vi "IE_Open Help Link.vi"(8 "error in (no error)":errorcluster, 11 "Help.URL":string) -> (0 "error out":errorcluster)   [LabVIEW 2021]
uses:
  <vilib>/Platform/browser.llb/Open URL in Default Browser (string).vi
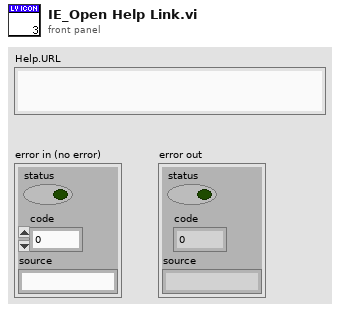
[diagram p1: front panel]
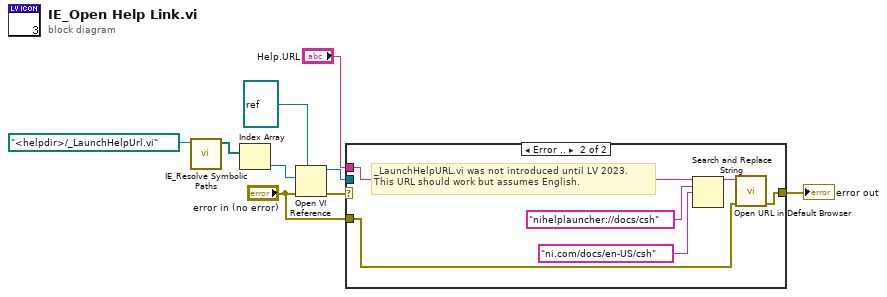
[diagram p0: block diagram]
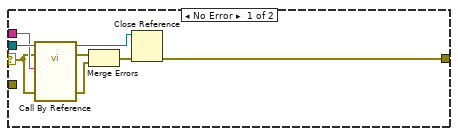
[diagram p2: hidden frame]
diagram:
  n1 = call "IE_Resolve Symbolic Paths.vi"("symbolic path"=path "<helpdir>/_LaunchHelpUrl.vi") -> ("resolved paths"=w8:path[])  [unwired: 10 in]
  n2 = Index Array(array=w8) -> (element=w7:path)  [unwired: 1 in]
  n3 = Open VI Reference(type specifier VI Refnum (for type only)=refnum<vi> refnum, vi path=w7, error in (no error)="error in (no error)") -> (vi reference=w6:refnum<vi>, error out=w3:errorcluster)  [unwired: 3 in]
  n4 = case shown="Error .." w3 {
    selector: w3 -> [w15 _]
    tunnel: w6 -> [w17 _]
    tunnel: "Help.URL" -> [w16 w20]
    tunnel: [w10 w23] -> w2
    tunnel: "error in (no error)" -> [_ w22]
    frame No Error {
      n5 = call-by-ref "?"(reference=w17, error in=w15, 4:"error in (no error)"=w15, "url"=w16) -> (reference out=w11:refnum<vi>, error out=w14:errorcluster, 0:"error out"=w13:errorcluster)  [unwired: 5 in]
      n6 = Merge Errors(w14, w13) -> (w12:errorcluster)
      n7 = Close Reference(reference=w11, error in (no error)=w12) -> (error out=w10:errorcluster)
    }
    frame Error {
      # "_LaunchHelpURL.vi was not introduced until LV 2023.\nThis URL should work but assumes English."
      n8 = Search and Replace String(input string=w20, search string="nihelplauncher://docs/csh", replace string="ni.com/docs/en-US/csh" ("replace string (\"\")")) -> (result string=w21:string)  [unwired: 5 in, 3 out]
      n9 = call-poly <vilib>:"Open URL in Default Browser.vi"("error in (no error)"=w22, "URL"=w21) -> ("error out"=w23:errorcluster)  [unwired: 4 in, 1 out]
    }
  }
  "error out" <- w2
